vi "PH_PPMA_PowerUnit.ProcState.vi"(0 "i ref in":refnum<vi>, 2 "state timeout":i32=-1, 4 "state":string, 5 "error in (no error)":errorcluster) -> (14 "i ref out":refnum<vi>, 18 "next state":string, 19 "error out":errorcluster)   [LabVIEW 2014, in "PH_PPMA_PowerUnit.lvlib"]
doc: "This VI represents part of the internal state machine of the object. All methods that are needed to implement the required functionality of the state machine will be called from THIS VI. Add your code here."
uses:
  PH_PPMA_PowerUnit.lvlib
  PH_PowerUnit_BaseClass/PH_PowerUnit_BaseClass.SM States.ctl
  CSCore/CSSystem/CoreDefs/CoreDefs.error_type.ctl
  CSCore/CSSystem/CoreLib/CoreLib.lvlib
  CSCore/BaseSM/BaseSM.lvlib
  PH_PSDBWriter/PH_PSDBWriter.lvlib
  PH_Beckhoff_PPMA-Rods/PH_Beckhoff_PPMA-Rods.lvlib
  PH_Beckhoff_PP_PU/PH_Beckhoff_PP_PU.lvlib
  PH_PowerUnit_BaseClass/PH_PowerUnit_BaseClass.lvlib
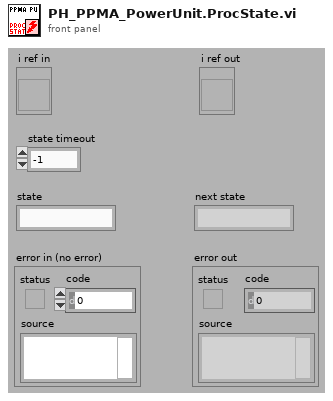
[diagram p1: front panel]
types:
  T1 = typedef "PH_PowerUnit_BaseClass.lvlib/PH_PowerUnit_BaseClass.SM States.ctl" = enum16{".", "Stand by", "Switch PU on", "Configure", "Set Default Voltage", "Set STANDBY", "Set READY", "Wait for Shot Cmd", "Open Dump Rods", "Open Ross Relais", "Close Ross Relais", "Switch PSU on", "Switch PSU off", "Charge", "Switch GD Channel on", "Close Dump Rods", "Rods-TO", "RR-TO", "PSU-TO", "Trigger-TO"}
  T2 = typedef "CoreDefs.error_type.ctl" = enum16{"no error", "can't load process", "can't unload process", "process does not exist", "can't install process", "can't remove process", "unknown function", "time out", "can't execute function", "duplicate queue name", "super not found", "caller queue invalid", "can't ping process", "unknown error", "VISA Error", "VISA timeout", "GPIB timeout", "GPIB error", "communication error", "data type mismatch", "can't read data from OPC server", "can't write data to OPC server", "OET error", "function not implemented", "process already exists", "invalid Shared Variable name", "error writing Shared Variable", "error reading Shared Variable", "invalid client name", "corrupt database", "unknown class", "call not authorized", "parameter out of range", "OET timeout: can't get data to modify", "invalid queue name", "requested operation incompatible with current state", "event undefined", "event disabled", "state undefined", "caller is not a friend", "EventBuilder: bad eventID", "EventBuilder: no DAQ devices", "a thread must not stop itself", "UNUSED ELEMENT4", "DiscArchiver: eventData incomplete", "DiscArchiver: eventData does not belong to run", "DiscArchiver: can't open file", "DiscArchiver: can't write to file", "DiscArchiver: available disc space low", "can't acquire semaphore", "error reading data from database", "notifier object is not existing", "can't register process", "can't unregister process", "illegal event type", "object disabled", "object already exists", "can't change state", "Instrument not found", "no connection to remote node", "invalid reference", "N/A", "UNUSED ELEMENT 1", "element not found", "illegal TCP/IP connection detected", "object does not exist", "invalid access ID", "unknown CS system", "invalid privilige", "unsupported data type", "unsupported server type", "IO server already exists", "Shared Variable already exists"}
  T3 = typedef "PH_PowerUnit_BaseClass.lvlib/PH_PowerUnit_BaseClass.i attribute.ctl" = cluster{"Constructor finished":bool, "PU":cluster{"In use":bool, "Service ID in use":i32, "GUI Ref":refnum<vi>}, "Enabling":cluster{"State":T4, "GUI Ref":refnum<vi>}, "Timing":cluster{"Last Shot":dbl, "Time between Shots [Sec]":dbl, "Waiting Time over?":bool, "Service ID Waiting Time":i32, "GUI Ref":refnum<vi>, "Instance":cluster{"Status":T5, "linked?":bool, "GUI Ref":refnum<vi>}}, "Sequencer":cluster{"SM State":string, "GUI Ref":refnum<vi>, "linked":bool}, "Subscribed Trendmssgs":cluster{"Tagname":string, "Status":T5, "linked?":bool, "Shot Condition":T5, "GUI Ref":refnum<vi>}[], "PP PU":T6, "Default Voltage (V)":dbl, "GUI Refs":T7, "PSDB data":cluster{"Shot Voltage [V]":dbl, "State TO SM":T1, "Write 2 early":bool}, "State TO SM":T1}
  T4 = typedef "PH_SystemInformation.lvlib/PH_SystemInformationEnabling State.ctl" = i32
  T5 = typedef "PH_StatusHandler.lvlib/PH_StatusHandler.Status.ctl" = i16
  T6 = typedef "PH_PP_Common.lvlib/PH_PP_Common.PUs.ctl" = enum16{"no Info", "PA-19mm-1", "PA-19mm-2", "PA-45mm-PILC", "PA-45mm-MAIN", "MA-PU-1", "MA-PU-2", "MA-PU-3", "MA-PU-4", "MA-PU-5", "MA-PU-6", "MA-FR", "MA-PILC", "PA-45mm-DP"}
  T7 = typedef "PH_PowerUnit_BaseClass.lvlib/PH_PowerUnit_BaseClass.GUI Refs.ctl" = cluster{"Delete Inst":refnum<vi>, "State TO SM":refnum<vi>, "State SM":refnum<vi>, "Fire":refnum<vi>}
  T8 = typedef "PH_PPMA_PowerUnit.lvlib/PH_PPMA_PowerUnit.i attribute.ctl" = cluster{"GUI Refs":cluster{"Rods":refnum<vi>, "Ignitron":refnum<vi>, "Rossrelais":refnum<vi>, "Set Voltage":refnum<vi>, "PSU":refnum<vi>, "EOC":refnum<vi>, "Trigger":refnum<vi>}, "Rods":T9, "PSU":T10, "Ross Relais":T11, "Ignitron":T12, "Trigger":cluster{"State Device":T5, "linked?":bool}, "Timing Settings":cluster{"Prdc Fast?":bool, "Default Value Periodic Interval":i32, "Mercury on since":dbl, "Warm up Time Mercury [s]":dbl}, "Set Voltage [V]":dbl}
  T9 = typedef "PH_PPMA_PowerUnit.lvlib/PH_PPMA_PowerUnit.Rods Attributes.ctl" = cluster{"Instancename":string, "Device Status":T5, "linked?":bool}
  T10 = typedef "PH_PP_Common.lvlib/PH_PP_Common.PSU Attributes.ctl" = cluster{"lower limit [V]":dbl, "upper limit [V]":dbl, "Voltage set":bool, "State Device":T5, "linked?":bool}
  T11 = typedef "PH_PP_Common.lvlib/PH_PP_Common.Ross Relais Attributes.ctl" = cluster{"State Device":T5, "linked?":bool}
  T12 = typedef "PH_PP_Common.lvlib/PH_PP_Common.Ignitron Attributes.ctl" = cluster{"State Device":T5, "linked?":bool}
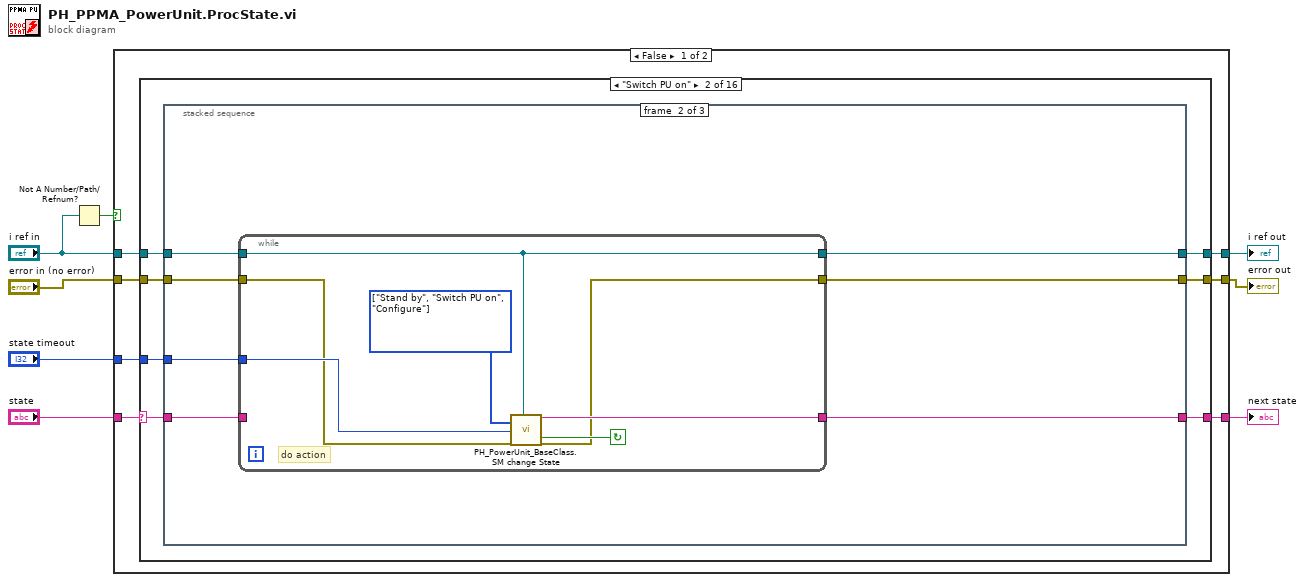
[diagram p0: block diagram]
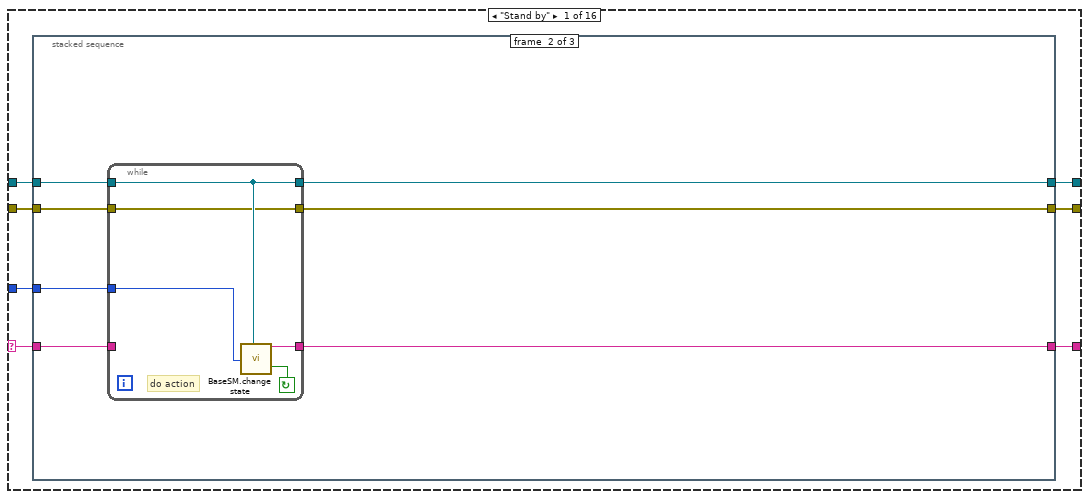
[diagram p2: hidden frame]
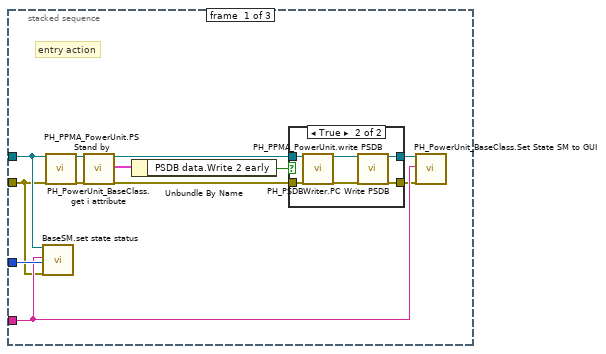
[diagram p3: hidden frame]
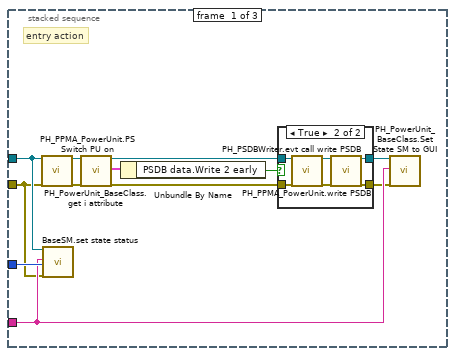
[diagram p6: hidden frame]
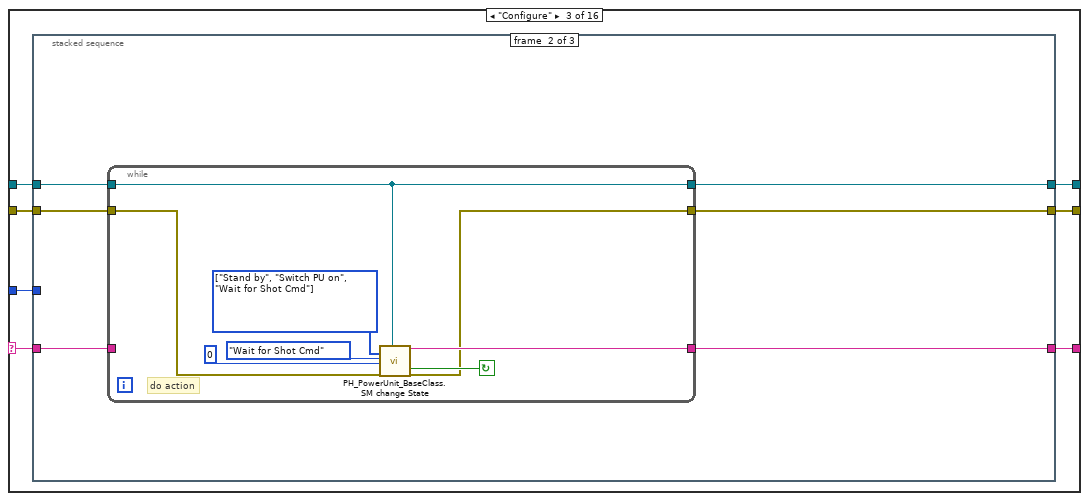
[diagram p9: hidden frame]
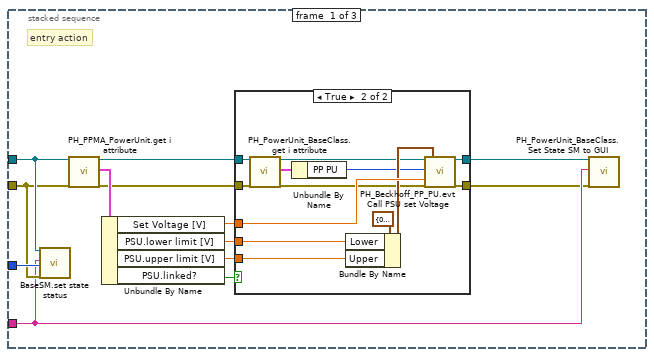
[diagram p10: hidden frame]
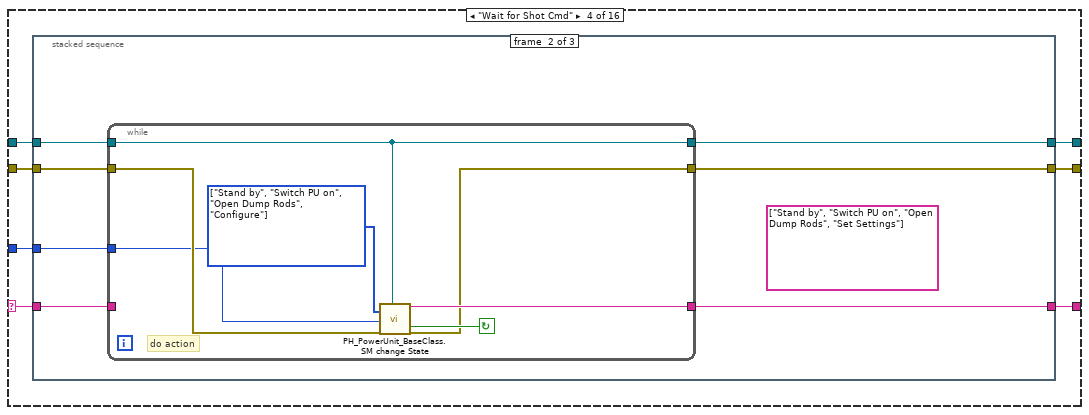
[diagram p13: hidden frame]
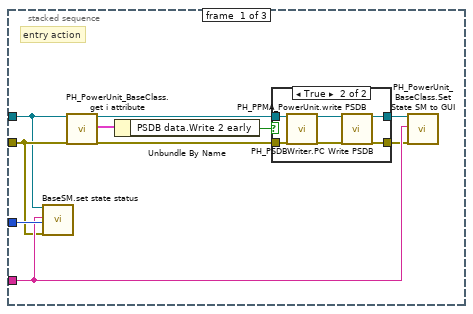
[diagram p14: hidden frame]
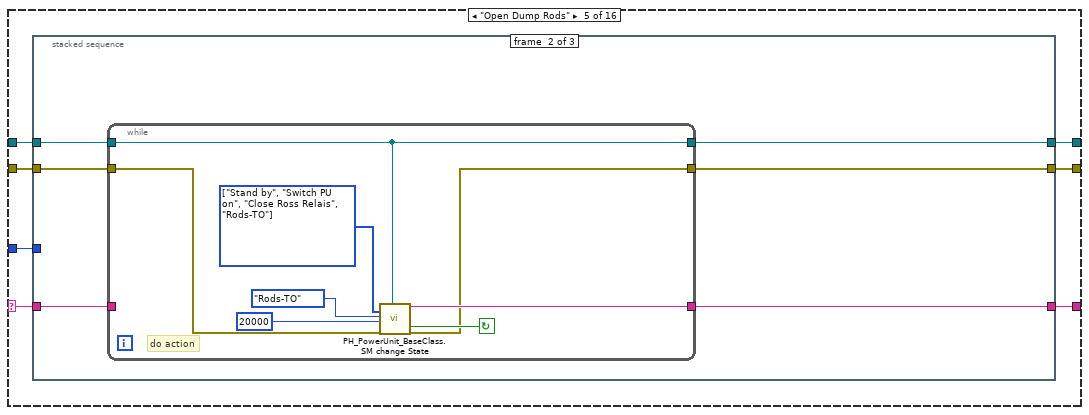
[diagram p17: hidden frame]
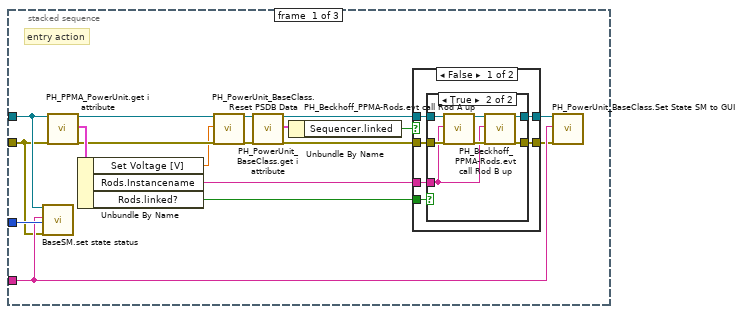
[diagram p18: hidden frame]
diagram:
  n1 = Not A Number/Path/Refnum?(number/path/refnum="i ref in") -> (NaN/Path/Refnum?=w2:bool)
  n2 = case shown="False" w2 {
    tunnel: "i ref in" -> [w15 w625]
    tunnel: [w14 w625] -> w8
    tunnel: "state" -> [w13 w622]
    tunnel: [w12 w622] -> w6
    tunnel: "state timeout" -> [w11 _]
    tunnel: "error in (no error)" -> [w10 _]
    tunnel: [w9 w623] -> w3
    frame False {
      n3 = case shown="\"Switch PU on\"" w13 {
        selector: w13 -> [w22 w61 w102 w151 w190 w246 w287 w349 w393 w435 w460 w513 w540 w567 w594 w616]
        tunnel: w15 -> [w20 w59 w100 w149 w188 w244 w285 w347 w391 w433 w458 w511 w538 w565 w592 w621]
        tunnel: [w19 w58 w99 w148 w187 w243 w284 w346 w390 w432 w457 w510 w537 w564 w591 w620] -> w14
        tunnel: [w21 w60 w101 w150 w189 w245 w286 w348 w392 w434 w459 w512 w539 w566 w593 w615] -> w12
        tunnel: w11 -> [w18 w57 w98 w147 w186 w242 w283 w345 w389 w431 w456 w509 w536 w563 w590 w617]
        tunnel: w10 -> [w17 w56 w97 w146 w185 w241 w282 w344 w388 w430 w455 w508 w535 w562 w589 w619]
        tunnel: [w16 w55 w96 w145 w184 w240 w281 w343 w387 w429 w454 w507 w534 w561 w588 w618] -> w9
        frame "Stand by" {
          n4 = stacked-sequence {
            tunnel: w22 -> [w33 w49 _]
            tunnel: [_ w48 _] -> w21
            tunnel: w20 -> [w32 w46 _]
            tunnel: [_ w45 _] -> w19
            tunnel: w18 -> [w34 w47 _]
            tunnel: w17 -> [w31 w43 _]
            tunnel: [_ w44 _] -> w16
            frame #0 {
              # "entry action"
              n5 = call "BaseSM.set state status.vi"("i ref in"=w32, "stateStatus"=w33, "ms timeout (10000)"=w34, "error in (no error)"=w31) -> ()  [unwired: 13 in, 3 out]
              n6 = call "PH_PPMA_PowerUnit.PS Stand by.vi"("i ref in"=w32, "error in (no error)"=w31) -> ("i ref out"=w26:refnum<vi>, "error out"=w25:errorcluster)  [unwired: 16 in]
              n7 = call "PH_PowerUnit_BaseClass.get i attribute.vi"("i ref in"=w26, "error in (no error)"=w25) -> ("i ref out"=w29:refnum<vi>, "i attribute"=w28:T3, "error out"=w30:errorcluster)  [unwired: 15 in]
              n8 = Unbundle By Name(w28) -> ("PSDB data.Write 2 early"=w27:bool)
              n9 = case shown="True" w27 {
                tunnel: w30 -> [w35 w37]
                tunnel: [w35 w39] -> w23
                tunnel: w29 -> [w36 w38]
                tunnel: [w36 w40] -> w24
                frame False {
                }
                frame True {
                  n10 = call "PH_PPMA_PowerUnit.write PSDB.vi"("i ref in"=w38, "error IO"=w37) -> ("i ref out"=w41:refnum<vi>, "error out"=w42:errorcluster)  [unwired: 16 in]
                  n11 = call "PH_PSDBWriter.PC Write PSDB.vi"("i ref in"=w41, "error IO"=w42) -> ("i ref out"=w40:refnum<vi>, "error out"=w39:errorcluster)  [unwired: 16 in]
                }
              }
              n12 = call "PH_PowerUnit_BaseClass.Set State SM to GUI.vi"("i ref in"=w24, "State SM"=w33, "error in (no error)"=w23) -> ()  [unwired: 15 in, 2 out]
            }
            frame #1 {
              n13 = while {
                tunnel: w47 -> [w52]
                tunnel: [w54] -> w48
                tunnel: w49 -> [_]
                tunnel: w46 -> [w51]
                tunnel: [w51] -> w45
                tunnel: [w50] -> w44
                tunnel: w43 -> [w50]
                stop <- w53 continue-if-true
                # "do action"
                n14 = call "BaseSM.change state.vi"("wait time [ms]"=w52, "i ref in"=w51) -> ("next state"=w54:string, "continue loop"=w53:bool)  [unwired: 14 in, 2 out]
              }
            }
            frame #2 {
              # "exit action"
            }
          }
        }
        frame "Switch PU on" {
          n15 = stacked-sequence {
            tunnel: w61 -> [w72 w88 _]
            tunnel: [_ w87 _] -> w60
            tunnel: w59 -> [w71 w85 _]
            tunnel: [_ w84 _] -> w58
            tunnel: w57 -> [w73 w86 _]
            tunnel: w56 -> [w70 w82 _]
            tunnel: [_ w83 _] -> w55
            frame #0 {
              # "entry action"
              n16 = call "PH_PPMA_PowerUnit.PS Switch PU on.vi"("i ref in"=w71, "error in (no error)"=w70) -> ("i ref out"=w63:refnum<vi>, "error out"=w62:errorcluster)  [unwired: 16 in]
              n17 = call "BaseSM.set state status.vi"("i ref in"=w71, "stateStatus"=w72, "ms timeout (10000)"=w73, "error in (no error)"=w70) -> ()  [unwired: 13 in, 3 out]
              n18 = call "PH_PowerUnit_BaseClass.get i attribute.vi"("i ref in"=w63, "error in (no error)"=w62) -> ("i ref out"=w68:refnum<vi>, "i attribute"=w67:T3, "error out"=w69:errorcluster)  [unwired: 15 in]
              n19 = Unbundle By Name(w67) -> ("PSDB data.Write 2 early"=w66:bool)
              n20 = case shown="True" w66 {
                tunnel: w69 -> [w74 w76]
                tunnel: [w74 w78] -> w64
                tunnel: w68 -> [w75 w77]
                tunnel: [w75 w79] -> w65
                frame False {
                }
                frame True {
                  n21 = call "PH_PPMA_PowerUnit.write PSDB.vi"("i ref in"=w77, "error IO"=w76) -> ("i ref out"=w80:refnum<vi>, "error out"=w81:errorcluster)  [unwired: 16 in]
                  n22 = call "PH_PSDBWriter.evt call write PSDB.vi"("i ref in"=w80, "error in (no error)"=w81) -> ("i ref out"=w79:refnum<vi>, "error out"=w78:errorcluster)  [unwired: 16 in]
                }
              }
              n23 = call "PH_PowerUnit_BaseClass.Set State SM to GUI.vi"("i ref in"=w65, "State SM"=w72, "error in (no error)"=w64) -> ()  [unwired: 15 in, 2 out]
            }
            frame #1 {
              n24 = while {
                tunnel: w86 -> [w93]
                tunnel: [w95] -> w87
                tunnel: w88 -> [_]
                tunnel: w85 -> [w92]
                tunnel: [w92] -> w84
                tunnel: [w90] -> w83
                tunnel: w82 -> [w91]
                stop <- w94 continue-if-true
                w89 = T1[] [enum."Stand by", enum."Switch PU on", enum."Configure"] items=[".", "Stand by", "Switch PU on", "Configure", "Set Default Voltage", "Set STANDBY", "Set READY", "Wait for Shot Cmd", "Open Dump Rods", "Open Ross Relais", "Close Ross Relais", "Switch PSU on", "Switch PSU off", "Charge", "Switch GD Channel on", "Close Dump Rods", "Rods-TO", "RR-TO", "PSU-TO", "Trigger-TO"] ("allowed next states")
                # "do action"
                n25 = call "PH_PowerUnit_BaseClass.SM change State.vi"("allowed next states"=w89, "wait time [ms]"=w93, "error in (no error)"=w91, "VI in"=w92) -> ("next state"=w95:string, "continue loop"=w94:bool, "error out"=w90:errorcluster)  [unwired: 13 in]
              }
            }
            frame #2 {
              # "exit action"
            }
          }
        }
        frame "Configure" {
          n26 = stacked-sequence {
            tunnel: w102 -> [w109 w136 _]
            tunnel: [_ w135 _] -> w101
            tunnel: w100 -> [w112 w134 _]
            tunnel: [_ w133 _] -> w99
            tunnel: w98 -> [w115 _ _]
            tunnel: w97 -> [w111 w131 _]
            tunnel: [_ w132 _] -> w96
            frame #0 {
              # "entry action"
              n27 = call "BaseSM.set state status.vi"("i ref in"=w112, "stateStatus"=w109, "ms timeout (10000)"=w115, "error in (no error)"=w111) -> ()  [unwired: 13 in, 3 out]
              n28 = call "PH_PPMA_PowerUnit.get i attribute.vi"("i ref in"=w112, "error in (no error)"=w111) -> ("i ref out"=w107:refnum<vi>, "i attribute"=w114:T8, "error out"=w110:errorcluster)  [unwired: 15 in]
              n29 = Unbundle By Name(w114) -> ("Set Voltage [V]"=w113:dbl, "PSU.lower limit [V]"=w106:dbl, "PSU.upper limit [V]"=w105:dbl, "PSU.linked?"=w108:bool)
              n30 = case shown="True" w108 {
                tunnel: w107 -> [w117 w119]
                tunnel: w110 -> [w116 w118]
                tunnel: w113 -> [_ w130]
                tunnel: [w116 w129] -> w103
                tunnel: [w117 w128] -> w104
                tunnel: w106 -> [_ w127]
                tunnel: w105 -> [_ w126]
                frame False {
                }
                frame True {
                  n31 = call "PH_PowerUnit_BaseClass.get i attribute.vi"("i ref in"=w119, "error in (no error)"=w118) -> ("i ref out"=w122:refnum<vi>, "i attribute"=w121:T3, "error out"=w123:errorcluster)  [unwired: 15 in]
                  n32 = Unbundle By Name(w121) -> ("PP PU"=w120:T6)
                  n33 = Bundle By Name(cluster=cluster{"Lower":dbl, "Upper":dbl} {"Lower"=0.0, "Upper"=0.0} ("Limits [V]"), "Lower"=w127, "Upper"=w126) -> (w124:cluster{"Lower":dbl, "Upper":dbl})
                  n34 = call "PH_Beckhoff_PP_PU.evt Call PSU set Voltage.vi"("i ref in"=w122, "PU"=w120, "Voltage to set [V]"=w130, "error in"=w123, "Limits [V]"=w124) -> ("i ref out"=w128:refnum<vi>, "error out"=w129:errorcluster)  [unwired: 13 in]
                }
              }
              n35 = call "PH_PowerUnit_BaseClass.Set State SM to GUI.vi"("i ref in"=w104, "State SM"=w109, "error in (no error)"=w103) -> ()  [unwired: 15 in, 2 out]
            }
            frame #1 {
              n36 = while {
                tunnel: [w144] -> w135
                tunnel: w136 -> [_]
                tunnel: w134 -> [w142]
                tunnel: [w142] -> w133
                tunnel: [w140] -> w132
                tunnel: w131 -> [w141]
                stop <- w143 continue-if-true
                w137 = T1[] [enum."Stand by", enum."Switch PU on", enum."Wait for Shot Cmd"] items=[".", "Stand by", "Switch PU on", "Configure", "Set Default Voltage", "Set STANDBY", "Set READY", "Wait for Shot Cmd", "Open Dump Rods", "Open Ross Relais", "Close Ross Relais", "Switch PSU on", "Switch PSU off", "Charge", "Switch GD Channel on", "Close Dump Rods", "Rods-TO", "RR-TO", "PSU-TO", "Trigger-TO"] ("allowed next states")
                # "do action"
                n37 = call "PH_PowerUnit_BaseClass.SM change State.vi"("allowed next states"=w137, "default state"=PH_PowerUnit_BaseClass.SM_States."Wait for Shot Cmd", "wait time [ms]"=0 ("wait time"), "error in (no error)"=w141, "VI in"=w142) -> ("next state"=w144:string, "continue loop"=w143:bool, "error out"=w140:errorcluster)  [unwired: 12 in]
              }
            }
            frame #2 {
              # "exit action"
            }
          }
        }
        frame "Wait for Shot Cmd" {
          n38 = stacked-sequence {
            tunnel: w151 -> [w160 w176 _]
            tunnel: [_ w175 _] -> w150
            tunnel: w149 -> [w157 w174 _]
            tunnel: [_ w173 _] -> w148
            tunnel: w147 -> [w161 w170 _]
            tunnel: w146 -> [w159 w171 _]
            tunnel: [_ w172 _] -> w145
            frame #0 {
              # "entry action"
              n39 = call "BaseSM.set state status.vi"("i ref in"=w157, "stateStatus"=w160, "ms timeout (10000)"=w161, "error in (no error)"=w159) -> ()  [unwired: 13 in, 3 out]
              n40 = call "PH_PowerUnit_BaseClass.get i attribute.vi"("i ref in"=w157, "error in (no error)"=w159) -> ("i ref out"=w156:refnum<vi>, "i attribute"=w155:T3, "error out"=w158:errorcluster)  [unwired: 15 in]
              n41 = Unbundle By Name(w155) -> ("PSDB data.Write 2 early"=w154:bool)
              n42 = case shown="True" w154 {
                tunnel: w158 -> [w162 w164]
                tunnel: [w162 w166] -> w152
                tunnel: w156 -> [w163 w165]
                tunnel: [w163 w167] -> w153
                frame False {
                }
                frame True {
                  n43 = call "PH_PPMA_PowerUnit.write PSDB.vi"("i ref in"=w165, "error IO"=w164) -> ("i ref out"=w168:refnum<vi>, "error out"=w169:errorcluster)  [unwired: 16 in]
                  n44 = call "PH_PSDBWriter.PC Write PSDB.vi"("i ref in"=w168, "error IO"=w169) -> ("i ref out"=w167:refnum<vi>, "error out"=w166:errorcluster)  [unwired: 16 in]
                }
              }
              n45 = call "PH_PowerUnit_BaseClass.Set State SM to GUI.vi"("i ref in"=w153, "State SM"=w160, "error in (no error)"=w152) -> ()  [unwired: 15 in, 2 out]
            }
            frame #1 {
              (unwired) string[] ["Stand by", "Switch PU on", "Open Dump Rods", "Set Settings"] ("allowed next states")
              n46 = while {
                tunnel: [w183] -> w175
                tunnel: w176 -> [_]
                tunnel: w174 -> [w181]
                tunnel: [w181] -> w173
                tunnel: [w179] -> w172
                tunnel: w171 -> [w180]
                tunnel: w170 -> [w178]
                stop <- w182 continue-if-true
                w177 = T1[] [enum."Stand by", enum."Switch PU on", enum."Open Dump Rods", enum."Configure"] items=[".", "Stand by", "Switch PU on", "Configure", "Set Default Voltage", "Set STANDBY", "Set READY", "Wait for Shot Cmd", "Open Dump Rods", "Open Ross Relais", "Close Ross Relais", "Switch PSU on", "Switch PSU off", "Charge", "Switch GD Channel on", "Close Dump Rods", "Rods-TO", "RR-TO", "PSU-TO", "Trigger-TO"] ("allowed next states")
                # "do action"
                n47 = call "PH_PowerUnit_BaseClass.SM change State.vi"("allowed next states"=w177, "wait time [ms]"=w178, "error in (no error)"=w180, "VI in"=w181) -> ("next state"=w183:string, "continue loop"=w182:bool, "error out"=w179:errorcluster)  [unwired: 13 in]
              }
            }
            frame #2 {
              # "exit action"
            }
          }
        }
        frame "Open Dump Rods" {
          n48 = stacked-sequence {
            tunnel: w190 -> [w206 w231 _]
            tunnel: [_ w230 _] -> w189
            tunnel: w188 -> [w199 w229 _]
            tunnel: [_ w228 _] -> w187
            tunnel: w186 -> [w208 _ _]
            tunnel: w185 -> [w198 w226 _]
            tunnel: [_ w227 _] -> w184
            frame #0 {
              # "entry action"
              n49 = call "BaseSM.set state status.vi"("i ref in"=w199, "stateStatus"=w206, "ms timeout (10000)"=w208, "error in (no error)"=w198) -> ()  [unwired: 13 in, 3 out]
              n50 = call "PH_PPMA_PowerUnit.get i attribute.vi"("i ref in"=w199, "error in (no error)"=w198) -> ("i ref out"=w197:refnum<vi>, "i attribute"=w204:T8, "error out"=w195:errorcluster)  [unwired: 15 in]
              n51 = Unbundle By Name(w204) -> ("Set Voltage [V]"=w193:dbl, "Rods.Instancename"=w207:string, "Rods.linked?"=w205:bool)
              n52 = call "PH_PowerUnit_BaseClass.Reset PSDB Data.vi"("VI in"=w197, "PSDB data.Shot Voltage [V]"=w193, "error in (no error)"=w195) -> ("VI out"=w196:refnum<vi>, "error out"=w194:errorcluster)  [unwired: 15 in]
              n53 = call "PH_PowerUnit_BaseClass.get i attribute.vi"("i ref in"=w196, "error in (no error)"=w194) -> ("i ref out"=w202:refnum<vi>, "i attribute"=w201:T3, "error out"=w203:errorcluster)  [unwired: 15 in]
              n54 = Unbundle By Name(w201) -> ("Sequencer.linked"=w200:bool)
              n55 = case shown="False" w200 {
                tunnel: w202 -> [w214 w224]
                tunnel: w203 -> [w213 w225]
                tunnel: w207 -> [w212 _]
                tunnel: [w211 w225] -> w191
                tunnel: [w210 w224] -> w192
                tunnel: w205 -> [w209 _]
                frame False {
                  n56 = case shown="True" w209 {
                    tunnel: w214 -> [w215 w223]
                    tunnel: w213 -> [w216 w222]
                    tunnel: w212 -> [_ w219]
                    tunnel: [w216 w220] -> w211
                    tunnel: [w215 w217] -> w210
                    frame False {
                    }
                    frame True {
                      n57 = call "PH_Beckhoff_PPMA-Rods.evt call Rod A up.vi"("i ref in"=w223, "Instance name"=w219, "error in"=w222) -> ("i ref out"=w218:refnum<vi>, "error out"=w221:errorcluster)  [unwired: 15 in]
                      n58 = call "PH_Beckhoff_PPMA-Rods.evt call Rod B up.vi"("i ref in"=w218, "Instance name"=w219, "error in"=w221) -> ("i ref out"=w217:refnum<vi>, "error out"=w220:errorcluster)  [unwired: 15 in]
                    }
                  }
                }
                frame True {
                }
              }
              n59 = call "PH_PowerUnit_BaseClass.Set State SM to GUI.vi"("i ref in"=w192, "State SM"=w206, "error in (no error)"=w191) -> ()  [unwired: 15 in, 2 out]
            }
            frame #1 {
              n60 = while {
                tunnel: [w239] -> w230
                tunnel: w231 -> [_]
                tunnel: w229 -> [w237]
                tunnel: [w237] -> w228
                tunnel: [w235] -> w227
                tunnel: w226 -> [w236]
                stop <- w238 continue-if-true
                w232 = T1[] [enum."Stand by", enum."Switch PU on", enum."Close Ross Relais", enum."Rods-TO"] items=[".", "Stand by", "Switch PU on", "Configure", "Set Default Voltage", "Set STANDBY", "Set READY", "Wait for Shot Cmd", "Open Dump Rods", "Open Ross Relais", "Close Ross Relais", "Switch PSU on", "Switch PSU off", "Charge", "Switch GD Channel on", "Close Dump Rods", "Rods-TO", "RR-TO", "PSU-TO", "Trigger-TO"] ("allowed next states")
                # "do action"
                n61 = call "PH_PowerUnit_BaseClass.SM change State.vi"("allowed next states"=w232, "default state"=PH_PowerUnit_BaseClass.SM_States."Rods-TO", "wait time [ms]"=20000 ("wait time"), "error in (no error)"=w236, "VI in"=w237) -> ("next state"=w239:string, "continue loop"=w238:bool, "error out"=w235:errorcluster)  [unwired: 12 in]
              }
            }
            frame #2 {
              # "exit action"
            }
          }
        }
        frame "Close Ross Relais" {
          n62 = stacked-sequence {
            tunnel: w246 -> [w250 w272 _]
            tunnel: [_ w271 _] -> w245
            tunnel: w244 -> [w252 w270 _]
            tunnel: [_ w269 _] -> w243
            tunnel: w242 -> [w256 _ _]
            tunnel: w241 -> [w251 w267 _]
            tunnel: [_ w268 _] -> w240
            frame #0 {
              # "entry action"
              n63 = call "BaseSM.set state status.vi"("i ref in"=w252, "stateStatus"=w250, "ms timeout (10000)"=w256, "error in (no error)"=w251) -> ()  [unwired: 13 in, 3 out]
              n64 = call "PH_PPMA_PowerUnit.get i attribute.vi"("i ref in"=w252, "error in (no error)"=w251) -> ("i ref out"=w254:refnum<vi>, "i attribute"=w255:T8, "error out"=w253:errorcluster)  [unwired: 15 in]
              n65 = Unbundle By Name(w255) -> ("Ross Relais.linked?"=w249:bool)
              n66 = case shown="True" w249 {
                tunnel: w254 -> [w257 w260]
                tunnel: w253 -> [w258 w259]
                tunnel: [w258 w266] -> w247
                tunnel: [w257 w265] -> w248
                frame False {
                }
                frame True {
                  n67 = call "PH_PowerUnit_BaseClass.get i attribute.vi"("i ref in"=w260, "error in (no error)"=w259) -> ("i ref out"=w263:refnum<vi>, "i attribute"=w262:T3, "error out"=w264:errorcluster)  [unwired: 15 in]
                  n68 = Unbundle By Name(w262) -> ("PP PU"=w261:T6)
                  n69 = call "PH_Beckhoff_PP_PU.evt Call RR close.vi"("i ref in"=w263, "PU"=w261, "error in"=w264) -> ("i ref out"=w265:refnum<vi>, "error out"=w266:errorcluster)  [unwired: 15 in]
                }
              }
              n70 = call "PH_PowerUnit_BaseClass.Set State SM to GUI.vi"("i ref in"=w248, "State SM"=w250, "error in (no error)"=w247) -> ()  [unwired: 15 in, 2 out]
            }
            frame #1 {
              n71 = while {
                tunnel: [w280] -> w271
                tunnel: w272 -> [_]
                tunnel: w270 -> [w278]
                tunnel: [w278] -> w269
                tunnel: [w276] -> w268
                tunnel: w267 -> [w277]
                stop <- w279 continue-if-true
                w273 = T1[] [enum."Stand by", enum."Switch PU on", enum."Switch PSU on", enum."RR-TO"] items=[".", "Stand by", "Switch PU on", "Configure", "Set Default Voltage", "Set STANDBY", "Set READY", "Wait for Shot Cmd", "Open Dump Rods", "Open Ross Relais", "Close Ross Relais", "Switch PSU on", "Switch PSU off", "Charge", "Switch GD Channel on", "Close Dump Rods", "Rods-TO", "RR-TO", "PSU-TO", "Trigger-TO"] ("allowed next states")
                # "do action"
                n72 = call "PH_PowerUnit_BaseClass.SM change State.vi"("allowed next states"=w273, "default state"=PH_PowerUnit_BaseClass.SM_States."RR-TO", "wait time [ms]"=20000 ("wait time"), "error in (no error)"=w277, "VI in"=w278) -> ("next state"=w280:string, "continue loop"=w279:bool, "error out"=w276:errorcluster)  [unwired: 12 in]
              }
            }
            frame #2 {
              # "exit action"
            }
          }
        }
        frame "Switch PSU on" {
          n73 = stacked-sequence {
            tunnel: w287 -> [w295 w334 _]
            tunnel: [_ w333 _] -> w286
            tunnel: w285 -> [w289 w332 _]
            tunnel: [_ w331 _] -> w284
            tunnel: w283 -> [w301 _ _]
            tunnel: w282 -> [w288 w329 _]
            tunnel: [_ w330 _] -> w281
            frame #0 {
              # "entry action"
              n74 = call "PH_PowerUnit_BaseClass.get i attribute.vi"("i ref in"=w289, "error in (no error)"=w288) -> ("i ref out"=w292:refnum<vi>, "i attribute"=w291:T3, "error out"=w293:errorcluster)  [unwired: 15 in]
              n75 = call "BaseSM.set state status.vi"("i ref in"=w289, "stateStatus"=w295, "ms timeout (10000)"=w301, "error in (no error)"=w288) -> ()  [unwired: 13 in, 3 out]
              n76 = Unbundle By Name(w291) -> ("PP PU"=w290:T6)
              n77 = call "PH_PPMA_PowerUnit.get i attribute.vi"("i ref in"=w292, "error in (no error)"=w293) -> ("i ref out"=w299:refnum<vi>, "i attribute"=w300:T8, "error out"=w298:errorcluster)  [unwired: 15 in]
              n78 = Unbundle By Name(w300) -> ("PSU.linked?"=w294:bool)
              n79 = case shown="True" w294 {
                tunnel: w299 -> [w302 w312]
                tunnel: w298 -> [w303 w311]
                tunnel: [w303 w313] -> w296
                tunnel: [w302 w314] -> w297
                tunnel: w290 -> [_ w310]
                frame False {
                }
                frame True {
                  n80 = flat-sequence {
                    tunnel: w312 -> [w319]
                    tunnel: w311 -> [w318]
                    tunnel: [w317] -> w309
                    tunnel: [w316] -> w308
                    tunnel: w310 -> [w315]
                    tunnel: [w315] -> w307
                    tunnel: w309 -> [w323]
                    tunnel: [w323] -> w306
                    tunnel: w308 -> [w322]
                    tunnel: [w322] -> w305
                    tunnel: w307 -> [w321]
                    tunnel: [w321] -> w304
                    tunnel: [w325] -> w313
                    tunnel: [w327] -> w314
                    tunnel: w306 -> [w328]
                    tunnel: w305 -> [w326]
                    tunnel: w304 -> [w324]
                    frame #0 {
                      n81 = call "PH_Beckhoff_PP_PU.evt Call PSU Inhibit off.vi"("i ref in"=w319, "PU"=w315, "error in"=w318) -> ("i ref out"=w317:refnum<vi>, "error out"=w316:errorcluster)  [unwired: 15 in]
                    }
                    frame #1 {
                      n82 = Wait (ms)(milliseconds to wait=u32 1000) -> ()  [unwired: 1 out]
                    }
                    frame #2 {
                      n83 = call "PH_Beckhoff_PP_PU.evt Call PSU HV on.vi"("i ref in"=w328, "PU"=w324, "error in"=w326) -> ("i ref out"=w327:refnum<vi>, "error out"=w325:errorcluster)  [unwired: 15 in]
                    }
                  }
                }
              }
              n84 = call "PH_PowerUnit_BaseClass.Set State SM to GUI.vi"("i ref in"=w297, "State SM"=w295, "error in (no error)"=w296) -> ()  [unwired: 15 in, 2 out]
            }
            frame #1 {
              n85 = while {
                tunnel: [w342] -> w333
                tunnel: w334 -> [_]
                tunnel: w332 -> [w340]
                tunnel: [w340] -> w331
                tunnel: [w338] -> w330
                tunnel: w329 -> [w339]
                stop <- w341 continue-if-true
                w335 = T1[] [enum."Stand by", enum."Switch PU on", enum."Switch PSU off", enum."PSU-TO"] items=[".", "Stand by", "Switch PU on", "Configure", "Set Default Voltage", "Set STANDBY", "Set READY", "Wait for Shot Cmd", "Open Dump Rods", "Open Ross Relais", "Close Ross Relais", "Switch PSU on", "Switch PSU off", "Charge", "Switch GD Channel on", "Close Dump Rods", "Rods-TO", "RR-TO", "PSU-TO", "Trigger-TO"] ("allowed next states")
                # "do action"
                n86 = call "PH_PowerUnit_BaseClass.SM change State.vi"("allowed next states"=w335, "default state"=PH_PowerUnit_BaseClass.SM_States."PSU-TO", "wait time [ms]"=60000 ("wait time"), "error in (no error)"=w339, "VI in"=w340) -> ("next state"=w342:string, "continue loop"=w341:bool, "error out"=w338:errorcluster)  [unwired: 12 in]
              }
            }
            frame #2 {
              # "exit action"
            }
          }
        }
        frame "Switch PSU off" {
          n87 = stacked-sequence {
            tunnel: w349 -> [w361 w378 _]
            tunnel: [_ w377 _] -> w348
            tunnel: w347 -> [w351 w376 _]
            tunnel: [_ w375 _] -> w346
            tunnel: w345 -> [w363 _ _]
            tunnel: w344 -> [w350 w373 _]
            tunnel: [_ w374 _] -> w343
            frame #0 {
              # "entry action"
              n88 = call "BaseSM.set state status.vi"("i ref in"=w351, "stateStatus"=w361, "ms timeout (10000)"=w363, "error in (no error)"=w350) -> ()  [unwired: 13 in, 3 out]
              n89 = call "PH_PowerUnit_BaseClass.get i attribute.vi"("i ref in"=w351, "error in (no error)"=w350) -> ("i ref out"=w354:refnum<vi>, "i attribute"=w353:T3, "error out"=w355:errorcluster)  [unwired: 15 in]
              n90 = Unbundle By Name(w353) -> ("PP PU"=w352:T6)
              n91 = call "PH_PPMA_PowerUnit.get i attribute.vi"("i ref in"=w354, "error in (no error)"=w355) -> ("i ref out"=w358:refnum<vi>, "i attribute"=w359:T8, "error out"=w357:errorcluster)  [unwired: 15 in]
              n92 = Unbundle By Name(w359) -> ("PSU.linked?"=w356:bool)
              n93 = case shown="True" w356 {
                tunnel: w358 -> [w364 w372]
                tunnel: w357 -> [w365 w371]
                tunnel: [w365 w368] -> w360
                tunnel: [w364 w367] -> w362
                tunnel: w352 -> [_ w366]
                frame False {
                }
                frame True {
                  n94 = call "PH_Beckhoff_PP_PU.evt Call PSU Inhibit on.vi"("i ref in"=w372, "PU"=w366, "error in"=w371) -> ("i ref out"=w370:refnum<vi>, "error out"=w369:errorcluster)  [unwired: 15 in]
                  n95 = call "PH_Beckhoff_PP_PU.evt Call PSU HV off.vi"("i ref in"=w370, "PU"=w366, "error in"=w369) -> ("i ref out"=w367:refnum<vi>, "error out"=w368:errorcluster)  [unwired: 15 in]
                }
              }
              n96 = call "PH_PowerUnit_BaseClass.Set State SM to GUI.vi"("i ref in"=w362, "State SM"=w361, "error in (no error)"=w360) -> ()  [unwired: 15 in, 2 out]
            }
            frame #1 {
              n97 = while {
                tunnel: [w386] -> w377
                tunnel: w378 -> [_]
                tunnel: w376 -> [w384]
                tunnel: [w384] -> w375
                tunnel: [w382] -> w374
                tunnel: w373 -> [w383]
                stop <- w385 continue-if-true
                w379 = T1[] [enum."Stand by", enum."Switch PU on", enum."Open Ross Relais", enum."PSU-TO"] items=[".", "Stand by", "Switch PU on", "Configure", "Set Default Voltage", "Set STANDBY", "Set READY", "Wait for Shot Cmd", "Open Dump Rods", "Open Ross Relais", "Close Ross Relais", "Switch PSU on", "Switch PSU off", "Charge", "Switch GD Channel on", "Close Dump Rods", "Rods-TO", "RR-TO", "PSU-TO", "Trigger-TO"] ("allowed next states")
                # "do action"
                n98 = call "PH_PowerUnit_BaseClass.SM change State.vi"("allowed next states"=w379, "default state"=PH_PowerUnit_BaseClass.SM_States."PSU-TO", "wait time [ms]"=10000 ("wait time"), "error in (no error)"=w383, "VI in"=w384) -> ("next state"=w386:string, "continue loop"=w385:bool, "error out"=w382:errorcluster)  [unwired: 12 in]
              }
            }
            frame #2 {
              # "exit action"
            }
          }
        }
        frame "Open Ross Relais" {
          n99 = stacked-sequence {
            tunnel: w393 -> [w404 w420 _]
            tunnel: [_ w419 _] -> w392
            tunnel: w391 -> [w394 w418 _]
            tunnel: [_ w417 _] -> w390
            tunnel: w389 -> [w407 _ _]
            tunnel: w388 -> [w395 w415 _]
            tunnel: [_ w416 _] -> w387
            frame #0 {
              # "entry action"
              n100 = call "BaseSM.set state status.vi"("i ref in"=w394, "stateStatus"=w404, "ms timeout (10000)"=w407, "error in (no error)"=w395) -> ()  [unwired: 13 in, 3 out]
              n101 = call "PH_PowerUnit_BaseClass.get i attribute.vi"("i ref in"=w394, "error in (no error)"=w395) -> ("i ref out"=w398:refnum<vi>, "i attribute"=w397:T3, "error out"=w399:errorcluster)  [unwired: 15 in]
              n102 = Unbundle By Name(w397) -> ("PP PU"=w396:T6)
              n103 = call "PH_PPMA_PowerUnit.get i attribute.vi"("i ref in"=w398, "error in (no error)"=w399) -> ("i ref out"=w402:refnum<vi>, "i attribute"=w403:T8, "error out"=w401:errorcluster)  [unwired: 15 in]
              n104 = Unbundle By Name(w403) -> ("Ross Relais.linked?"=w400:bool)
              n105 = case shown="True" w400 {
                tunnel: w402 -> [w408 w414]
                tunnel: w401 -> [w409 w413]
                tunnel: [w409 w412] -> w405
                tunnel: [w408 w411] -> w406
                tunnel: w396 -> [_ w410]
                frame False {
                }
                frame True {
                  n106 = call "PH_Beckhoff_PP_PU.evt Call RR open.vi"("i ref in"=w414, "PU"=w410, "error in"=w413) -> ("i ref out"=w411:refnum<vi>, "error out"=w412:errorcluster)  [unwired: 15 in]
                }
              }
              n107 = call "PH_PowerUnit_BaseClass.Set State SM to GUI.vi"("i ref in"=w406, "State SM"=w404, "error in (no error)"=w405) -> ()  [unwired: 15 in, 2 out]
            }
            frame #1 {
              n108 = while {
                tunnel: [w428] -> w419
                tunnel: w420 -> [_]
                tunnel: w418 -> [w426]
                tunnel: [w426] -> w417
                tunnel: [w424] -> w416
                tunnel: w415 -> [w425]
                stop <- w427 continue-if-true
                w421 = T1[] [enum."Stand by", enum."Switch PU on", enum."Switch GD Channel on", enum."RR-TO"] items=[".", "Stand by", "Switch PU on", "Configure", "Set Default Voltage", "Set STANDBY", "Set READY", "Wait for Shot Cmd", "Open Dump Rods", "Open Ross Relais", "Close Ross Relais", "Switch PSU on", "Switch PSU off", "Charge", "Switch GD Channel on", "Close Dump Rods", "Rods-TO", "RR-TO", "PSU-TO", "Trigger-TO"] ("allowed next states")
                # "do action"
                n109 = call "PH_PowerUnit_BaseClass.SM change State.vi"("allowed next states"=w421, "default state"=PH_PowerUnit_BaseClass.SM_States."RR-TO", "wait time [ms]"=10000 ("wait time"), "error in (no error)"=w425, "VI in"=w426) -> ("next state"=w428:string, "continue loop"=w427:bool, "error out"=w424:errorcluster)  [unwired: 12 in]
              }
            }
            frame #2 {
              # "exit action"
            }
          }
        }
        frame "Switch GD Channel on" {
          n110 = stacked-sequence {
            tunnel: w435 -> [w438 w445 _]
            tunnel: [_ w444 _] -> w434
            tunnel: w433 -> [w437 w443 _]
            tunnel: [_ w442 _] -> w432
            tunnel: w431 -> [w439 _ _]
            tunnel: w430 -> [w436 w440 _]
            tunnel: [_ w441 _] -> w429
            frame #0 {
              # "entry action"
              n111 = call "BaseSM.set state status.vi"("i ref in"=w437, "stateStatus"=w438, "ms timeout (10000)"=w439, "error in (no error)"=w436) -> ()  [unwired: 13 in, 3 out]
              n112 = call "PH_PowerUnit_BaseClass.Set State SM to GUI.vi"("i ref in"=w437, "State SM"=w438, "error in (no error)"=w436) -> ()  [unwired: 15 in, 2 out]
            }
            frame #1 {
              n113 = while {
                tunnel: [w453] -> w444
                tunnel: w445 -> [_]
                tunnel: w443 -> [w448]
                tunnel: [w448] -> w442
                tunnel: [w451] -> w441
                tunnel: w440 -> [w449]
                stop <- w452 continue-if-true
                w446 = T1[] [enum."Stand by", enum."Switch PU on", enum."Close Dump Rods", enum."Trigger-TO"] items=[".", "Stand by", "Switch PU on", "Configure", "Set Default Voltage", "Set STANDBY", "Set READY", "Wait for Shot Cmd", "Open Dump Rods", "Open Ross Relais", "Close Ross Relais", "Switch PSU on", "Switch PSU off", "Charge", "Switch GD Channel on", "Close Dump Rods", "Rods-TO", "RR-TO", "PSU-TO", "Trigger-TO"] ("allowed next states")
                # "do action"
                n114 = call "PH_PowerUnit_BaseClass.SM change State.vi"("allowed next states"=w446, "default state"=PH_PowerUnit_BaseClass.SM_States."Trigger-TO", "wait time [ms]"=60000, "error in (no error)"=w449, "VI in"=w448) -> ("next state"=w453:string, "continue loop"=w452:bool, "error out"=w451:errorcluster)  [unwired: 12 in]
              }
            }
            frame #2 {
              # "exit action"
            }
          }
        }
        frame "Close Dump Rods" {
          n115 = stacked-sequence {
            tunnel: w460 -> [w470 w498 _]
            tunnel: [_ w497 _] -> w459
            tunnel: w458 -> [w472 w496 _]
            tunnel: [_ w495 _] -> w457
            tunnel: w456 -> [w475 _ _]
            tunnel: w455 -> [w471 w493 _]
            tunnel: [_ w494 _] -> w454
            frame #0 {
              # "entry action"
              n116 = call "PH_PPMA_PowerUnit.get i attribute.vi"("i ref in"=w472, "error in (no error)"=w471) -> ("i ref out"=w466:refnum<vi>, "i attribute"=w474:T8, "error out"=w468:errorcluster)  [unwired: 15 in]
              n117 = call "BaseSM.set state status.vi"("i ref in"=w472, "stateStatus"=w470, "ms timeout (10000)"=w475, "error in (no error)"=w471) -> ()  [unwired: 13 in, 3 out]
              n118 = Unbundle By Name(w474) -> ("Rods.Instancename"=w473:string, "Rods.linked?"=w469:bool)
              n119 = call "PH_PowerUnit_BaseClass.get i attribute.vi"("i ref in"=w466, "error in (no error)"=w468) -> ("i ref out"=w465:refnum<vi>, "i attribute"=w464:T3, "error out"=w467:errorcluster)  [unwired: 15 in]
              n120 = Unbundle By Name(w464) -> ("Sequencer.linked"=w463:bool)
              n121 = case shown="False" w463 {
                tunnel: w465 -> [w481 w491]
                tunnel: w467 -> [w480 w492]
                tunnel: w473 -> [w479 _]
                tunnel: [w477 w492] -> w461
                tunnel: [w476 w491] -> w462
                tunnel: w469 -> [w478 _]
                frame False {
                  n122 = case shown="True" w478 {
                    tunnel: w481 -> [w483 w490]
                    tunnel: w480 -> [w482 w489]
                    tunnel: [w483 w485] -> w476
                    tunnel: [w482 w487] -> w477
                    tunnel: w479 -> [_ w484]
                    frame False {
                    }
                    frame True {
                      n123 = call "PH_Beckhoff_PPMA-Rods.evt call Rod A down.vi"("i ref in"=w490, "Instance name"=w484, "error in"=w489) -> ("i ref out"=w486:refnum<vi>, "error out"=w488:errorcluster)  [unwired: 15 in]
                      n124 = call "PH_Beckhoff_PPMA-Rods.evt call Rod B down.vi"("i ref in"=w486, "Instance name"=w484, "error in"=w488) -> ("i ref out"=w485:refnum<vi>, "error out"=w487:errorcluster)  [unwired: 15 in]
                    }
                  }
                }
                frame True {
                }
              }
              n125 = call "PH_PowerUnit_BaseClass.Set State SM to GUI.vi"("i ref in"=w462, "State SM"=w470, "error in (no error)"=w461) -> ()  [unwired: 15 in, 2 out]
            }
            frame #1 {
              n126 = while {
                tunnel: [w506] -> w497
                tunnel: w498 -> [_]
                tunnel: w496 -> [w502]
                tunnel: [w502] -> w495
                tunnel: [w504] -> w494
                tunnel: w493 -> [w503]
                stop <- w505 continue-if-true
                w499 = T1[] [enum."Stand by", enum."Switch PU on", enum."Wait for Shot Cmd", enum."Rods-TO"] items=[".", "Stand by", "Switch PU on", "Configure", "Set Default Voltage", "Set STANDBY", "Set READY", "Wait for Shot Cmd", "Open Dump Rods", "Open Ross Relais", "Close Ross Relais", "Switch PSU on", "Switch PSU off", "Charge", "Switch GD Channel on", "Close Dump Rods", "Rods-TO", "RR-TO", "PSU-TO", "Trigger-TO"] ("allowed next states")
                # "do action"
                n127 = call "PH_PowerUnit_BaseClass.SM change State.vi"("allowed next states"=w499, "default state"=PH_PowerUnit_BaseClass.SM_States."Rods-TO", "wait time [ms]"=10000 ("wait time"), "error in (no error)"=w503, "VI in"=w502) -> ("next state"=w506:string, "continue loop"=w505:bool, "error out"=w504:errorcluster)  [unwired: 12 in]
              }
            }
            frame #2 {
              # "exit action"
            }
          }
        }
        frame "Rods-TO" {
          n128 = stacked-sequence {
            tunnel: w513 -> [w516 w525 _]
            tunnel: [_ w524 _] -> w512
            tunnel: w511 -> [w515 w523 _]
            tunnel: [_ w522 _] -> w510
            tunnel: w509 -> [w519 _ _]
            tunnel: w508 -> [w514 w520 _]
            tunnel: [_ w521 _] -> w507
            frame #0 {
              # "entry action"
              n129 = call "BaseSM.set state status.vi"("i ref in"=w515, "stateStatus"=w516, "ms timeout (10000)"=w519, "error in (no error)"=w514) -> ()  [unwired: 13 in, 3 out]
              n130 = call "PH_PowerUnit_BaseClass.handle TO.vi"("VI in"=w515, "String"=w516, "error in (no error)"=w514) -> ("VI out"=w518:refnum<vi>, "error out"=w517:errorcluster)  [unwired: 15 in]
              n131 = call "PH_PowerUnit_BaseClass.Set State SM to GUI.vi"("i ref in"=w518, "State SM"=w516, "error in (no error)"=w517) -> ()  [unwired: 15 in, 2 out]
            }
            frame #1 {
              n132 = while {
                tunnel: [w533] -> w524
                tunnel: w525 -> [_]
                tunnel: w523 -> [w529]
                tunnel: [w529] -> w522
                tunnel: [w531] -> w521
                tunnel: w520 -> [w530]
                stop <- w532 continue-if-true
                w526 = T1[] [enum."Stand by", enum."Switch PU on"] items=[".", "Stand by", "Switch PU on", "Configure", "Set Default Voltage", "Set STANDBY", "Set READY", "Wait for Shot Cmd", "Open Dump Rods", "Open Ross Relais", "Close Ross Relais", "Switch PSU on", "Switch PSU off", "Charge", "Switch GD Channel on", "Close Dump Rods", "Rods-TO", "RR-TO", "PSU-TO", "Trigger-TO"] ("allowed next states")
                # "do action"
                n133 = call "PH_PowerUnit_BaseClass.SM change State.vi"("allowed next states"=w526, "default state"=PH_PowerUnit_BaseClass.SM_States."Switch PU on", "wait time [ms]"=0 ("wait time"), "error in (no error)"=w530, "VI in"=w529) -> ("next state"=w533:string, "continue loop"=w532:bool, "error out"=w531:errorcluster)  [unwired: 12 in]
              }
            }
            frame #2 {
              # "exit action"
            }
          }
        }
        frame "RR-TO" {
          n134 = stacked-sequence {
            tunnel: w540 -> [w545 w552 _]
            tunnel: [_ w551 _] -> w539
            tunnel: w538 -> [w542 w550 _]
            tunnel: [_ w549 _] -> w537
            tunnel: w536 -> [w546 _ _]
            tunnel: w535 -> [w541 w547 _]
            tunnel: [_ w548 _] -> w534
            frame #0 {
              # "entry action"
              n135 = call "BaseSM.set state status.vi"("i ref in"=w542, "stateStatus"=w545, "ms timeout (10000)"=w546, "error in (no error)"=w541) -> ()  [unwired: 13 in, 3 out]
              n136 = call "PH_PowerUnit_BaseClass.handle TO.vi"("VI in"=w542, "String"=w545, "error in (no error)"=w541) -> ("VI out"=w544:refnum<vi>, "error out"=w543:errorcluster)  [unwired: 15 in]
              n137 = call "PH_PowerUnit_BaseClass.Set State SM to GUI.vi"("i ref in"=w544, "State SM"=w545, "error in (no error)"=w543) -> ()  [unwired: 15 in, 2 out]
            }
            frame #1 {
              n138 = while {
                tunnel: [w560] -> w551
                tunnel: w552 -> [_]
                tunnel: w550 -> [w556]
                tunnel: [w556] -> w549
                tunnel: [w558] -> w548
                tunnel: w547 -> [w557]
                stop <- w559 continue-if-true
                w553 = T1[] [enum."Stand by", enum."Switch PU on"] items=[".", "Stand by", "Switch PU on", "Configure", "Set Default Voltage", "Set STANDBY", "Set READY", "Wait for Shot Cmd", "Open Dump Rods", "Open Ross Relais", "Close Ross Relais", "Switch PSU on", "Switch PSU off", "Charge", "Switch GD Channel on", "Close Dump Rods", "Rods-TO", "RR-TO", "PSU-TO", "Trigger-TO"] ("allowed next states")
                # "do action"
                n139 = call "PH_PowerUnit_BaseClass.SM change State.vi"("allowed next states"=w553, "default state"=PH_PowerUnit_BaseClass.SM_States."Switch PU on", "wait time [ms]"=0 ("wait time"), "error in (no error)"=w557, "VI in"=w556) -> ("next state"=w560:string, "continue loop"=w559:bool, "error out"=w558:errorcluster)  [unwired: 12 in]
              }
            }
            frame #2 {
              # "exit action"
            }
          }
        }
        frame "PSU-TO" {
          n140 = stacked-sequence {
            tunnel: w567 -> [w572 w579 _]
            tunnel: [_ w578 _] -> w566
            tunnel: w565 -> [w569 w577 _]
            tunnel: [_ w576 _] -> w564
            tunnel: w563 -> [w573 _ _]
            tunnel: w562 -> [w568 w574 _]
            tunnel: [_ w575 _] -> w561
            frame #0 {
              # "entry action"
              n141 = call "BaseSM.set state status.vi"("i ref in"=w569, "stateStatus"=w572, "ms timeout (10000)"=w573, "error in (no error)"=w568) -> ()  [unwired: 13 in, 3 out]
              n142 = call "PH_PowerUnit_BaseClass.handle TO.vi"("VI in"=w569, "String"=w572, "error in (no error)"=w568) -> ("VI out"=w571:refnum<vi>, "error out"=w570:errorcluster)  [unwired: 15 in]
              n143 = call "PH_PowerUnit_BaseClass.Set State SM to GUI.vi"("i ref in"=w571, "State SM"=w572, "error in (no error)"=w570) -> ()  [unwired: 15 in, 2 out]
            }
            frame #1 {
              n144 = while {
                tunnel: [w587] -> w578
                tunnel: w579 -> [_]
                tunnel: w577 -> [w583]
                tunnel: [w583] -> w576
                tunnel: [w585] -> w575
                tunnel: w574 -> [w584]
                stop <- w586 continue-if-true
                w580 = T1[] [enum."Stand by", enum."Switch PU on"] items=[".", "Stand by", "Switch PU on", "Configure", "Set Default Voltage", "Set STANDBY", "Set READY", "Wait for Shot Cmd", "Open Dump Rods", "Open Ross Relais", "Close Ross Relais", "Switch PSU on", "Switch PSU off", "Charge", "Switch GD Channel on", "Close Dump Rods", "Rods-TO", "RR-TO", "PSU-TO", "Trigger-TO"] ("allowed next states")
                # "do action"
                n145 = call "PH_PowerUnit_BaseClass.SM change State.vi"("allowed next states"=w580, "default state"=PH_PowerUnit_BaseClass.SM_States."Switch PU on", "wait time [ms]"=0 ("wait time"), "error in (no error)"=w584, "VI in"=w583) -> ("next state"=w587:string, "continue loop"=w586:bool, "error out"=w585:errorcluster)  [unwired: 12 in]
              }
            }
            frame #2 {
              # "exit action"
            }
          }
        }
        frame "Trigger-TO" {
          n146 = stacked-sequence {
            tunnel: w594 -> [w599 w606 _]
            tunnel: [_ w605 _] -> w593
            tunnel: w592 -> [w596 w604 _]
            tunnel: [_ w603 _] -> w591
            tunnel: w590 -> [w600 _ _]
            tunnel: w589 -> [w595 w601 _]
            tunnel: [_ w602 _] -> w588
            frame #0 {
              # "entry action"
              n147 = call "BaseSM.set state status.vi"("i ref in"=w596, "stateStatus"=w599, "ms timeout (10000)"=w600, "error in (no error)"=w595) -> ()  [unwired: 13 in, 3 out]
              n148 = call "PH_PowerUnit_BaseClass.handle TO.vi"("VI in"=w596, "String"=w599, "error in (no error)"=w595) -> ("VI out"=w598:refnum<vi>, "error out"=w597:errorcluster)  [unwired: 15 in]
              n149 = call "PH_PowerUnit_BaseClass.Set State SM to GUI.vi"("i ref in"=w598, "State SM"=w599, "error in (no error)"=w597) -> ()  [unwired: 15 in, 2 out]
            }
            frame #1 {
              n150 = while {
                tunnel: [w614] -> w605
                tunnel: w606 -> [_]
                tunnel: w604 -> [w610]
                tunnel: [w610] -> w603
                tunnel: [w612] -> w602
                tunnel: w601 -> [w611]
                stop <- w613 continue-if-true
                w607 = T1[] [enum."Stand by", enum."Switch PU on"] items=[".", "Stand by", "Switch PU on", "Configure", "Set Default Voltage", "Set STANDBY", "Set READY", "Wait for Shot Cmd", "Open Dump Rods", "Open Ross Relais", "Close Ross Relais", "Switch PSU on", "Switch PSU off", "Charge", "Switch GD Channel on", "Close Dump Rods", "Rods-TO", "RR-TO", "PSU-TO", "Trigger-TO"] ("allowed next states")
                # "do action"
                n151 = call "PH_PowerUnit_BaseClass.SM change State.vi"("allowed next states"=w607, "default state"=PH_PowerUnit_BaseClass.SM_States."Switch PU on", "wait time [ms]"=0 ("wait time"), "error in (no error)"=w611, "VI in"=w610) -> ("next state"=w614:string, "continue loop"=w613:bool, "error out"=w612:errorcluster)  [unwired: 12 in]
              }
            }
            frame #2 {
              # "exit action"
            }
          }
        }
        frame Default {
          n152 = call "BaseSM.ProcState.vi"("i ref in"=w621, "state timeout [ms]"=w617, "state"=w616, "error in (no error)"=w619) -> ("i ref out"=w620:refnum<vi>, "next state"=w615:string, "error out"=w618:errorcluster)  [unwired: 13 in]
        }
      }
    }
    frame True {
      n153 = call "CoreLib.my to LV error.vi"("ErrorTypes"=CoreDefs.error_type."invalid reference") -> ("myErrorCluster"=w623:errorcluster)  [unwired: 17 in, 1 out]
    }
  }
  "i ref out" <- w8
  "next state" <- w6
  "error out" <- w3
